vi "chart add series on axis.vi"(7 "y_axis":u32, 8 "error in (no error)":errorcluster, 9 "values":string, 10 "categories":string, 11 "chart":u32) -> (0 "error out":errorcluster, 3 "function return":u32)   [LabVIEW 2015, in "xlsxwriter.lvlib"]
doc: "lxw_chart_series chart_add_series_on_axis(lxw_chart chart, const char *categories, const char *values, lxw_chart_axis y_axis);"
uses:
  xlsxwriter.lvlib
  xlsxwriter.dll
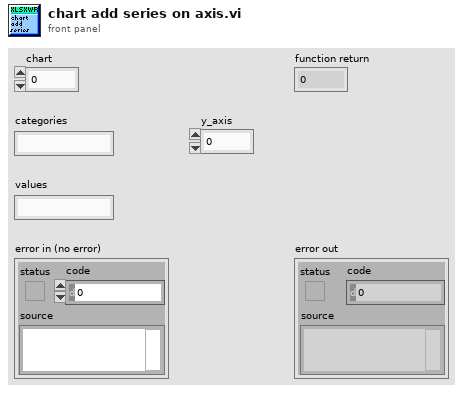
[diagram p1: front panel]
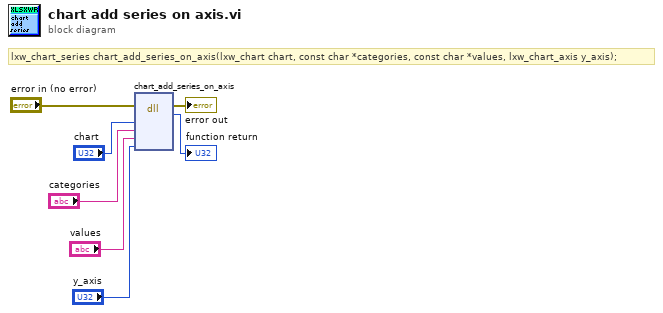
[diagram p0: block diagram]
diagram:
  # "lxw_chart_series chart_add_series_on_axis(lxw_chart chart, const char *categories, const char *values, lxw_chart_axis y_axis);"
  n1 = dll-call lib="C:/Users/WDAGUtilityAccount/Desktop/lv_vis_added_cell/xlsxwriter.*" fn="chart_add_series_on_axis"(error in="error in (no error)", "chart"="chart", "categories"="categories", "values"="values", "y_axis"="y_axis") -> (error out=→"error out":errorcluster, →"function return":u32)  [unwired: 6 in, 1 out]
